vi "HtmlPrepareHugo.vi"(6 "Additional Description":string, 8 "error in":errorcluster, 9 "ViTitle":string, 10 "ViDescr":string, 11 "Html Path":path) -> (0 "error out":errorcluster)   [LabVIEW 2020]
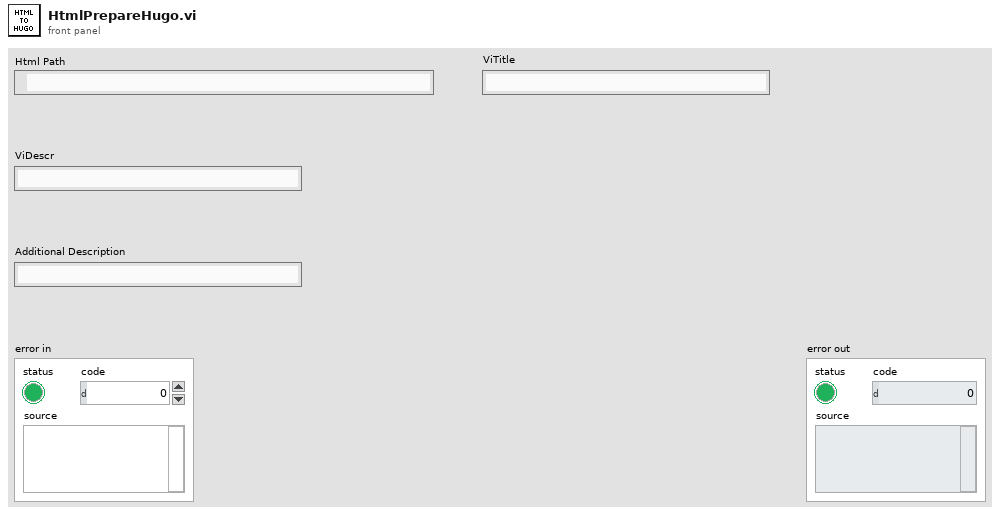
[diagram p1: front panel]
types:
  T1 = enum16{"open", "replace", "create", "open or create", "replace or create", "replace or create with confirmation"}
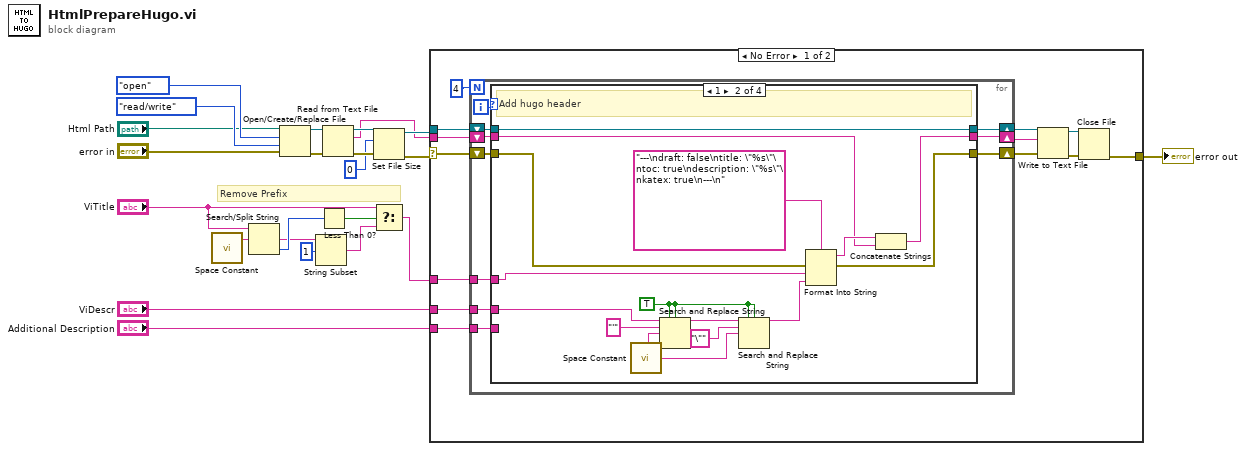
[diagram p0: block diagram]
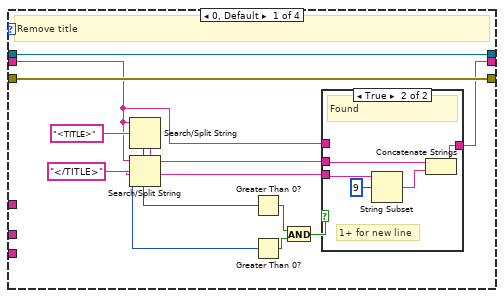
[diagram p2: hidden frame]
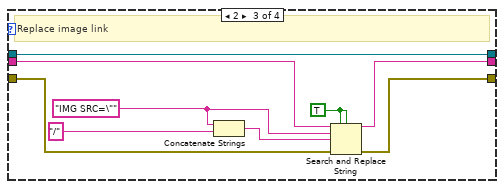
[diagram p4: hidden frame]
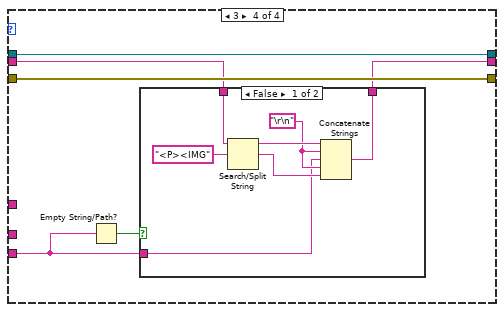
[diagram p5: hidden frame]
diagram:
  # "Remove Prefix"
  n1 = call <vilib>:"Space Constant.vi"() -> ("String"=w5:string)
  n2 = Search/Split String(string="ViTitle", search string/char (-)=w5) -> (match + rest of string=w4:string, offset of match=w9:i32)  [unwired: 1 in, 1 out]
  n3 = Open/Create/Replace File(file path (use dialog)="Html Path", error in="error in", operation (0:open)=T1."open", access (0:read/write)=enum16{"read/write", "read-only", "write-only"}."read/write") -> (refnum out=w21:refnum<file>, error out=w22:errorcluster)  [unwired: 2 in, 1 out]
  n4 = String Subset(string=w4, offset (0)=1) -> (substring=w8:string)  [unwired: 1 in]
  n5 = Less Than 0?(x=w9) -> (x < 0?=w7:bool)
  n6 = Read from Text File(file (use dialog)=w21, error in=w22) -> (refnum out=w17:refnum<file>, text=w13:string, error out=w18:errorcluster)  [unwired: 2 in, 1 out]
  n7 = Set File Size(4:w18, 6:i64 0 ("size (in bytes)"), 7:w17) -> (0:w15:errorcluster, 3:w16:refnum<file>)
  n8 = Select(t="ViTitle", s=w7, f=w8) -> (s? t:f=w6:string)
  n9 = case shown="No Error" w15 {
    selector: w15 -> [w33 w104]
    tunnel: w13 -> [w36 _]
    tunnel: w16 -> [w34 _]
    tunnel: [w28 w104] -> w23
    tunnel: "ViDescr" -> [w25 _]
    tunnel: w6 -> [w26 _]
    tunnel: "Additional Description" -> [w24 _]
    frame No Error {
      n10 = for {
        N: 4 -> [_]
        shift-right: [w40] -> w31
        shift-left: w33 -> [w41]
        shift-right: [w44] -> w27
        shift-left: w34 -> [w45]
        shift-right: [w42] -> w32
        shift-left: w36 -> [w43]
        tunnel: w26 -> [w39]
        tunnel: w25 -> [w38]
        tunnel: w24 -> [w37]
        i -> [w46]
        # "remove title"
        n11 = case shown="1" w46 {
          tunnel: w45 -> [w59 w80 w89 w95]
          tunnel: [w59 w80 w89 w95] -> w44
          tunnel: w43 -> [w48 w76 w86 w93]
          tunnel: [w47 w79 w85 w92] -> w42
          tunnel: w41 -> [w56 w74 w88 w94]
          tunnel: [w56 w73 w87 w94] -> w40
          tunnel: w38 -> [_ w71 _ _]
          tunnel: w39 -> [_ w66 _ _]
          tunnel: w37 -> [_ _ _ w91]
          frame 0, Default {
            # "Remove title"
            n12 = Search/Split String(string=w48, search string/char (-)="<TITLE>") -> (substring before match=w50:string, offset of match=w52:i32)  [unwired: 1 in, 1 out]
            n13 = Search/Split String(string=w48, search string/char (-)="</TITLE>") -> (match + rest of string=w49:string, offset of match=w53:i32)  [unwired: 1 in, 1 out]
            n14 = Greater Than 0?(x=w52) -> (x > 0?=w58:bool)
            n15 = Greater Than 0?(x=w53) -> (x > 0?=w57:bool)
            n16 = And(x=w58, y=w57) -> (x .and. y?=w51:bool)
            n17 = case shown="True" w51 {
              tunnel: w50 -> [_ w63]
              tunnel: w49 -> [_ w65]
              tunnel: w48 -> [w60 _]
              tunnel: [w60 w61] -> w47
              frame False {
                # "not found"
              }
              frame True {
                # "1+ for new line"
                # "Found"
                n18 = String Subset(string=w65, offset (0)=9) -> (substring=w62:string)  [unwired: 1 in]
                n19 = Concatenate Strings(w63, w62) -> (w61:string)
              }
            }
          }
          frame 1 {
            w68 = TRUE
            # "Add hugo header"
            n20 = call <vilib>:"Space Constant.vi"() -> ("String"=w69:string)
            n21 = Search and Replace String(replace all?=w68, case sensitive?=w68, input string=w71, search string="'", replace string=w69) -> (result string=w72:string)  [unwired: 3 in, 3 out]
            n22 = Search and Replace String(replace all?=w68, case sensitive?=w68, input string=w72, search string="\"", replace string=w69) -> (result string=w67:string)  [unwired: 3 in, 3 out]
            n23 = Format Into String(format string="---\ndraft: false\ntitle: \"%s\"\ntoc: true\ndescription: \"%s\"\nkatex: true\n---\n", error in=w74, w66, w67) -> (resulting string=w77:string, error out=w73:errorcluster)  [unwired: 1 in]
            n24 = Concatenate Strings(w77, w76) -> (w79:string)
          }
          frame 2 {
            w84 = TRUE
            w81 = "IMG SRC=\""
            # "Replace image link"
            n25 = Concatenate Strings(w81, "/") -> (w82:string)
            n26 = Search and Replace String(replace all?=w84, case sensitive?=w84, input string=w86, search string=w81, replace string=w82, error in=w88) -> (result string=w85:string, error out=w87:errorcluster)  [unwired: 2 in, 2 out]
          }
          frame 3 {
            n27 = Empty String/Path?(string/path=w91) -> (empty?=w90:bool)
            n28 = case shown="False" w90 {
              tunnel: w93 -> [w101 w103]
              tunnel: [w98 w103] -> w92
              tunnel: w91 -> [w96 _]
              frame False {
                w97 = "\r\n"
                n29 = Search/Split String(string=w101, search string/char (-)="<P><IMG") -> (substring before match=w100:string, match + rest of string=w99:string)  [unwired: 1 in, 1 out]
                n30 = Concatenate Strings(w100, w97, w96, w97, w99) -> (w98:string)
              }
              frame True {
              }
            }
          }
        }
      }
      n31 = Write to Text File(file (use dialog)=w27, text=w32, error in=w31) -> (refnum out=w29:refnum<file>, error out=w30:errorcluster)  [unwired: 1 in, 1 out]
      n32 = Close File(refnum=w29, error in=w30) -> (error out=w28:errorcluster)  [unwired: 1 out]
    }
    frame Error {
    }
  }
  "error out" <- w23
